vi "quick.vi"(10 "簇":T1, 11 "字符串":string) -> ()   [LabVIEW 2018]
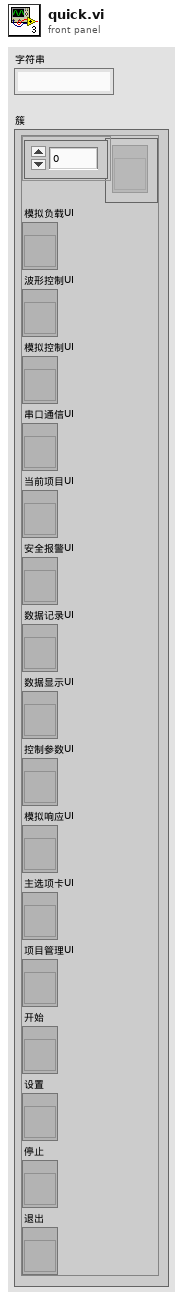
[diagram p1: front panel]
types:
  T1 = typedef "引用簇.ctl" = cluster{"数组":refnum<vi>[], "模拟负载UI":refnum<vi>, "波形控制UI":refnum<vi>, "模拟控制UI":refnum<vi>, "串口通信UI":refnum<vi>, "当前项目UI":refnum<vi>, "安全报警UI":refnum<vi>, "数据记录UI":refnum<vi>, "数据显示UI":refnum<vi>, "控制参数UI":refnum<vi>, "模拟响应UI":refnum<vi>, "主选项卡UI":refnum<vi>, "项目管理UI":refnum<vi>, "开始":refnum<vi>, "设置":refnum<vi>, "停止":refnum<vi>, "退出":refnum<vi>}
  T2 = enum32{"开始页", "当前项目配置", "串口通信配置", "控制参数配置", "模拟响应配置", "模拟控制配置", "模拟负载配置", "安全报警配置", "数据显示配置", "数据记录配置", "波形输出1", "波形输出2", "波形输出3", "波形输出4", "波形输出5", "波形输出6"}
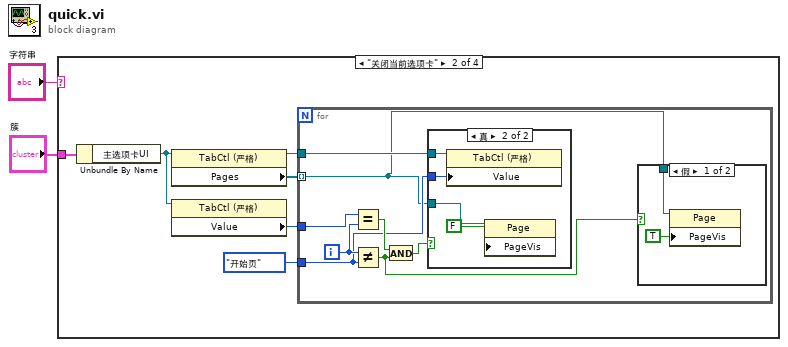
[diagram p0: block diagram]
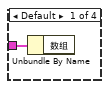
[diagram p2: hidden frame]
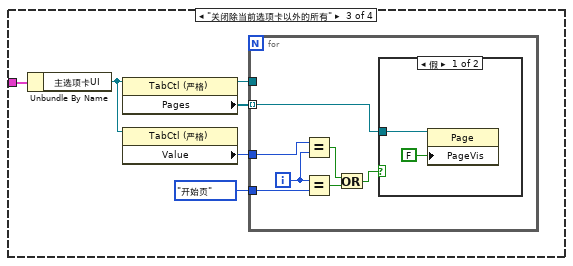
[diagram p5: hidden frame]
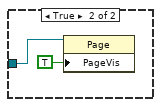
[diagram p6: hidden frame]
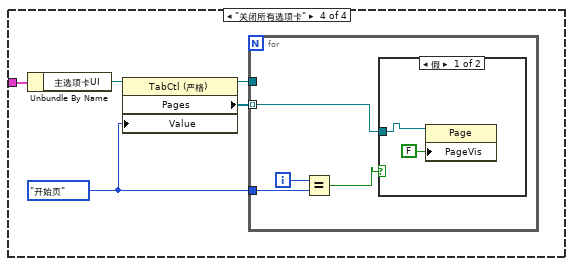
[diagram p7: hidden frame]
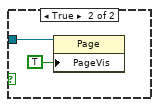
[diagram p8: hidden frame]
diagram:
  n1 = case shown="\"关闭当前选项卡\"" "字符串" {
    tunnel: "簇" -> [w3 w9 w29 w45]
    frame Default {
      n2 = Unbundle By Name(w3) -> ()  [unwired: 1 out]
    }
    frame "关闭当前选项卡" {
      n3 = Unbundle By Name(w9) -> ("主选项卡UI"=w8:refnum<vi>)
      n4 = property class="TabCtl (严格)"(reference=w8) -> (reference out=w5:refnum<vi>, "Pages"=w6:refnum<vi>[])  [unwired: 1 in, 1 out]
      n5 = property class="TabCtl (严格)"(reference=w8) -> ("Value"=w7:T2)  [unwired: 1 in, 2 out]
      n6 = for {
        tunnel: w7 -> [w17]
        tunnel: w6 -> [w10] mode=indexing
        tunnel: w5 -> [w13]
        tunnel: T2."开始页" ("值") -> [w12]
        i -> [w16]
        n7 = Equal?(x=w17, y=w16) -> (x = y?=w15:bool)
        n8 = Not Equal?(x=w16, y=w12) -> (x != y?=w11:bool)
        n9 = And(x=w15, y=w11) -> (x .and. y?=w14:bool)
        n10 = case shown="真" w14 {
          tunnel: w10 -> [_ w22]
          tunnel: w13 -> [_ w21]
          tunnel: w12 -> [_ w20]
          frame False {
          }
          frame True {
            n11 = property class="TabCtl (严格)"(reference=w21, "Value"=w20) -> ()  [unwired: 1 in, 2 out]
            n12 = property class="Page"(reference=w22, "PageVis"=FALSE ("选项卡可见")) -> ()  [unwired: 1 in, 2 out]
          }
        }
        n13 = case shown="假" w11 {
          tunnel: w10 -> [w18 _]
          frame False {
            n14 = property class="Page"(reference=w18, "PageVis"=TRUE ("选项卡可见")) -> ()  [unwired: 1 in, 2 out]
          }
          frame True {
          }
        }
      }
    }
    frame "关闭除当前选项卡以外的所有" {
      n15 = Unbundle By Name(w29) -> ("主选项卡UI"=w28:refnum<vi>)
      n16 = property class="TabCtl (严格)"(reference=w28) -> (reference out=w25:refnum<vi>, "Pages"=w26:refnum<vi>[])  [unwired: 1 in, 1 out]
      n17 = property class="TabCtl (严格)"(reference=w28) -> ("Value"=w27:T2)  [unwired: 1 in, 2 out]
      n18 = for {
        tunnel: w27 -> [w36]
        tunnel: w26 -> [w35] mode=indexing
        tunnel: w25 -> [_]
        tunnel: T2."开始页" ("值") -> [w30]
        i -> [w34]
        n19 = Equal?(x=w36, y=w34) -> (x = y?=w33:bool)
        n20 = Equal?(x=w34, y=w30) -> (x = y?=w32:bool)
        n21 = Or(x=w33, y=w32) -> (x .or. y?=w31:bool)
        n22 = case shown="假" w31 {
          tunnel: w35 -> [w37 w39]
          frame False {
            n23 = property class="Page"(reference=w37, "PageVis"=FALSE ("选项卡可见")) -> ()  [unwired: 1 in, 2 out]
          }
          frame True {
            n24 = property class="Page"(reference=w39, "PageVis"=TRUE ("选项卡可见")) -> ()  [unwired: 1 in, 2 out]
          }
        }
      }
    }
    frame "关闭所有选项卡" {
      w41 = T2."开始页" ("值")
      n25 = Unbundle By Name(w45) -> ("主选项卡UI"=w42:refnum<vi>)
      n26 = property class="TabCtl (严格)"(reference=w42, "Value"=w41) -> (reference out=w43:refnum<vi>, "Pages"=w44:refnum<vi>[])  [unwired: 1 in, 1 out]
      n27 = for {
        tunnel: w44 -> [w49] mode=indexing
        tunnel: w43 -> [_]
        tunnel: w41 -> [w47]
        i -> [w48]
        n28 = Equal?(x=w48, y=w47) -> (x = y?=w46:bool)
        n29 = case shown="假" w46 {
          tunnel: w49 -> [w51 w52]
          frame False {
            n30 = property class="Page"(reference=w51, "PageVis"=FALSE ("选项卡可见")) -> ()  [unwired: 1 in, 2 out]
          }
          frame True {
            n31 = property class="Page"(reference=w52, "PageVis"=TRUE ("选项卡可见")) -> ()  [unwired: 1 in, 2 out]
          }
        }
      }
    }
  }
